vi "Check Expansion Chassis Present.vi"(4 "error in":errorcluster, 5 "Timeout (60000ms)":u32=60000, 7 "IPs":string[](array[string])) -> (0 "error out":errorcluster, 1 "Timeout?":bool, 2 "Timeout Time (ms)":u32, 3 "Present?":bool[](array[boolean]))   [LabVIEW 2018, in "Outputs.lvlib"]
uses:
  Outputs.lvlib
  <vilib>/nisyscfg/Close (System).vi
  <vilib>/nisyscfg/nisyscfg.lvlib
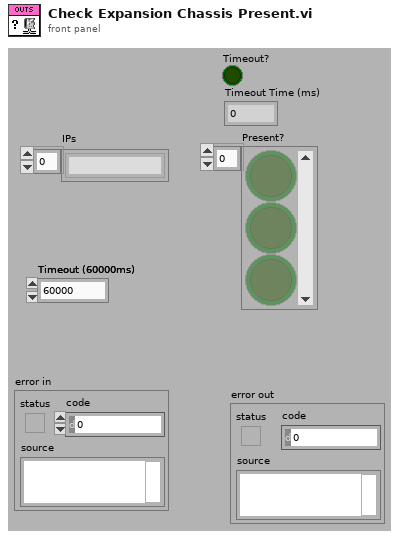
[diagram p1: front panel]
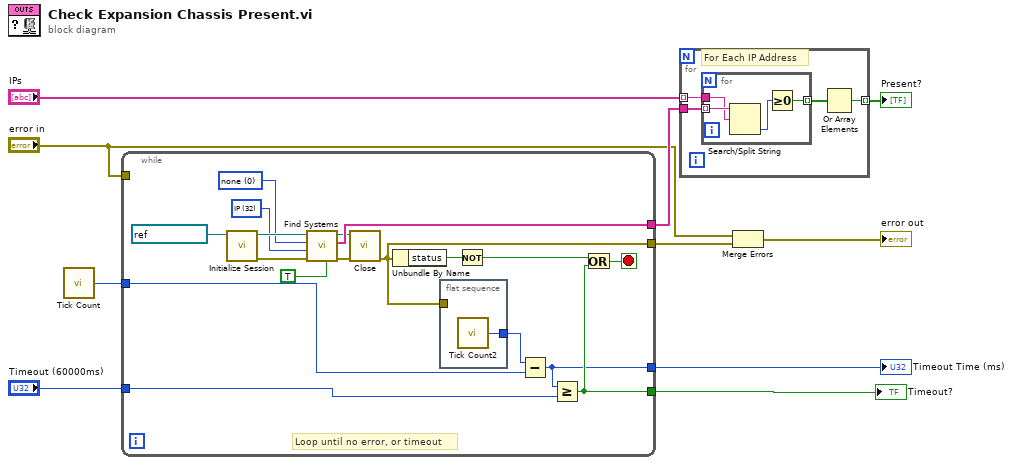
[diagram p0: block diagram]
diagram:
  n1 = call "Tick Count"() -> ("Tick Count(mSec)"=w5:u32)
  n2 = while {
    tunnel: [w28] -> w8
    tunnel: "error in" -> [_]
    tunnel: [w11] -> w7
    tunnel: w5 -> [w15]
    tunnel: "Timeout (60000ms)" -> [w14]
    tunnel: [w13] -> w3
    tunnel: [w12] -> w1
    stop <- w17 stop-if-true
    w21 = u32 0 items=["none"=0, "only if online"=1, "all"=3] ("Include Cached Results (all)")
    w22 = u32 32 items=["Hostname"=16, "Hostname (IP)"=18, "Hostname (MAC)"=19, "IP"=32, "IP (Hostname)"=33, "IP (MAC)"=35, "MAC"=48, "MAC (Hostname)"=49, "MAC (IP)"=50] ("Output (Hostname and IP)")
    # "Loop until no error, or timeout"
    n3 = call <vilib>:"Initialize Session.vi"("Target (localhost)"=refnum<k21> "localhost") -> ("error out"=w26:errorcluster, "Session out"=w25:refnum<k21>)  [unwired: 9 in]
    n4 = call <vilib>:"Find Systems.vi"("Only Installable Systems (F)"=TRUE, "error in (no error)"=w26, "Output (Hostname and IP)"=w22, "Include Cached Results (all)"=w21, "Session in (localhost)"=w25) -> ("error out"=w23:errorcluster, "Detected Systems"=w28:string[], "Session out"=w24:refnum<k21>)  [unwired: 4 in]
    n5 = call-poly <vilib>:"Close.vi"("error in (no error)"=w23, "Session in"=w24) -> ("error out"=w11:errorcluster)  [unwired: 9 in]
    n6 = Unbundle By Name(w11) -> ("status"=w19:bool)
    n7 = flat-sequence {
      tunnel: [w29] -> w16
      tunnel: w11 -> [_]
      frame #0 {
        n8 = call "Tick Count2"() -> ("Tick Count(mSec)"=w29:u32)
      }
    }
    n9 = Not(x=w19) -> (.not. x?=w18:bool)
    n10 = Subtract(x=w16, y=w15) -> (x-y=w12:u32)
    n11 = Greater Or Equal?(x=w12, y=w14) -> (x >= y?=w13:bool)
    n12 = Or(x=w18, y=w13) -> (x .or. y?=w17:bool)
  }
  "Timeout?" <- w3
  "Timeout Time (ms)" <- w1
  n13 = for {
    tunnel: w8 -> [w33]
    tunnel: [w31] -> w10 mode=indexing
    tunnel: "IPs" -> [w30] mode=indexing
    # "For Each IP Address"
    n14 = for {
      tunnel: w33 -> [w37] mode=indexing
      tunnel: w30 -> [w36]
      tunnel: [w34] -> w32 mode=indexing
      n15 = Search/Split String(string=w37, search string/char (-)=w36) -> (offset of match=w35:i32)  [unwired: 1 in, 2 out]
      n16 = Greater Or Equal To 0?(x=w35) -> (x >= 0?=w34:bool)
    }
    n17 = Or Array Elements(Boolean array=w32) -> (logical OR=w31:bool)
  }
  "Present?" <- w10
  n18 = Merge Errors("error in", w7) -> (→"error out":errorcluster)
